vi "Sensor X Facade.vi"(0 "Data In":T5, 2 "Display State In":T3, 3 "Container State":T4) -> (6 "Data Out":T5, 7 "Display State Out":T3, 8 "Action":T2)   [LabVIEW 2013, in "Sensor X.xctl"]
uses:
  Sensor X.xctl
  Sensor X Data.ctl
  lib/Data Access Objects/Sensors/Sensor DAO Class.lvclass
  <vilib>/_xctls/Container State.ctl
  Sensor X State.ctl
  <vilib>/_xctls/Action.ctl
  Sensor Metadata.ctl
  lib/Data Access Objects/Sensors/Sensor DAO Class.lvclass/Sensor DAO Class.ctl
  <vilib>/_xctls/XControlSupport.lvlib
panel:
  in  "Sensor Metadata":T1
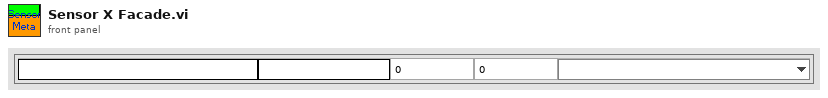
[diagram p1: front panel]
types:
  T1 = typedef "Sensor Metadata.ctl" = cluster{"Name":string, "Units":string, "Sensitivity":dbl, "Multiplier":dbl, "Excitation":u16}
  T2 = typedef "XControlSupport.lvlib/Action.ctl" = cluster{"Data Changed?":bool, "State Changed?":bool, "Action Name":string}
  T3 = typedef "Sensor X.xctl/Sensor X State.ctl" = cluster{"Volt Channels":string[]}
  T4 = typedef "XControlSupport.lvlib/Container State.ctl" = cluster{"Indicator?":bool, "Run Mode?":bool, " Refnum":refnum<vi>}
  T5 = typedef "Sensor X.xctl/Sensor X Data.ctl" = refnum<class "Sensor DAO Class.lvclass">
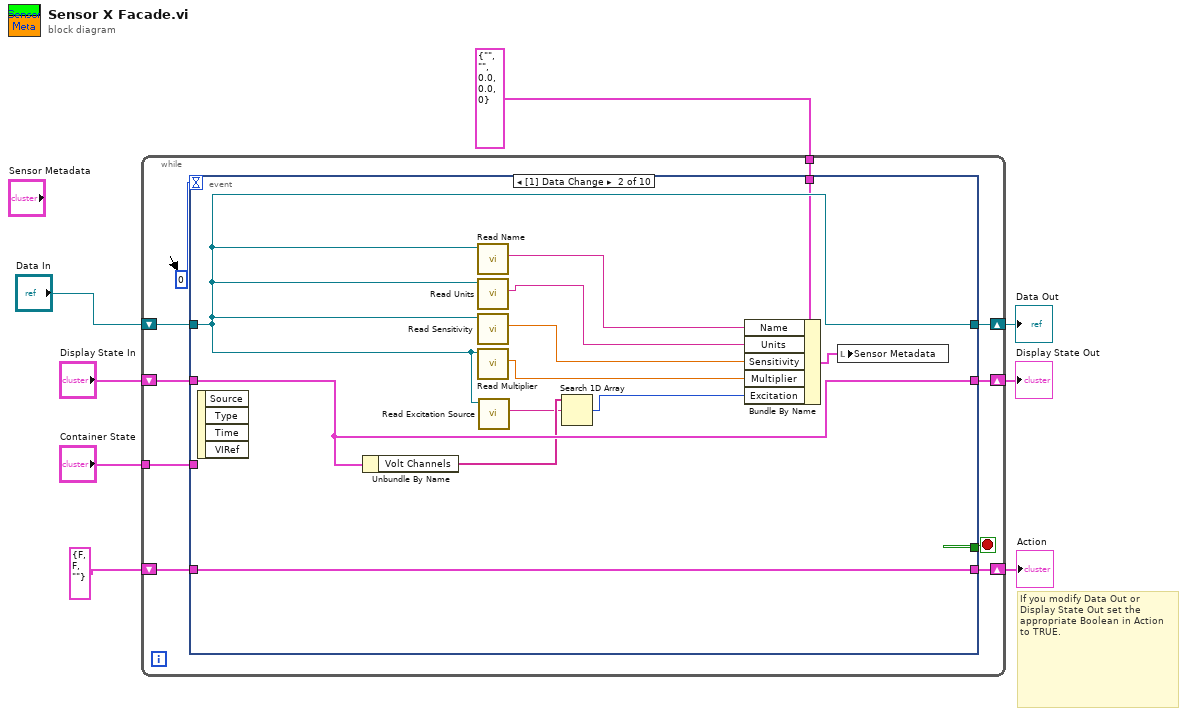
[diagram p0: block diagram]
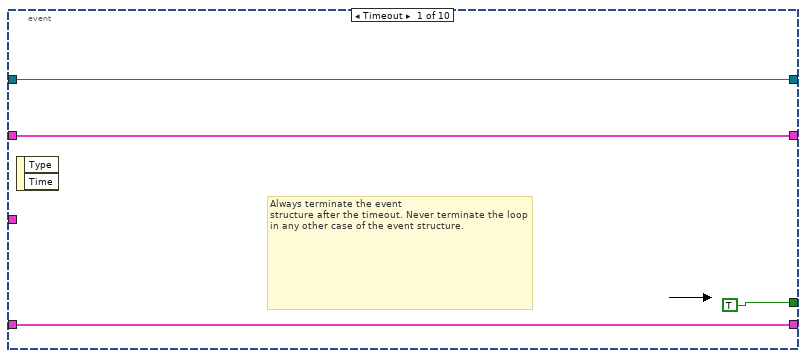
[diagram p2: hidden frame]
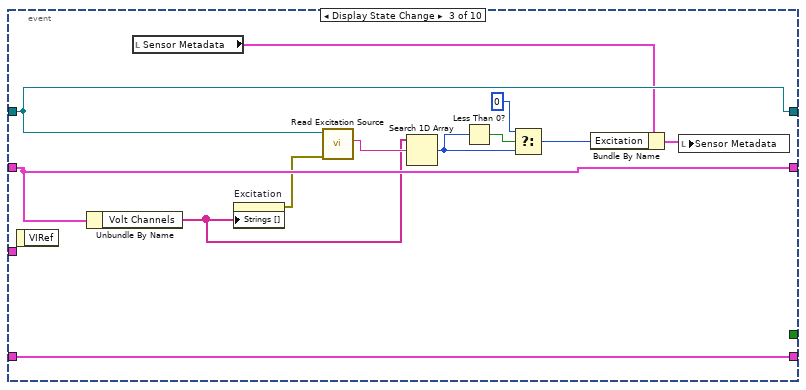
[diagram p3: hidden frame]
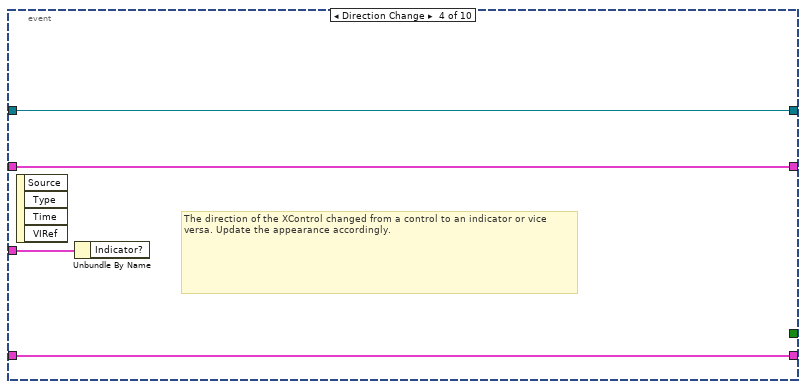
[diagram p4: hidden frame]
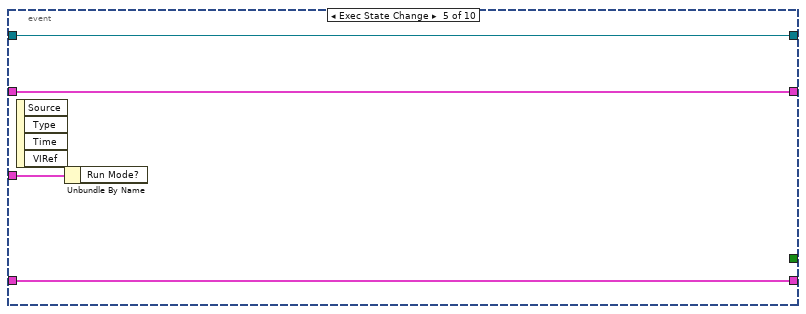
[diagram p5: hidden frame]
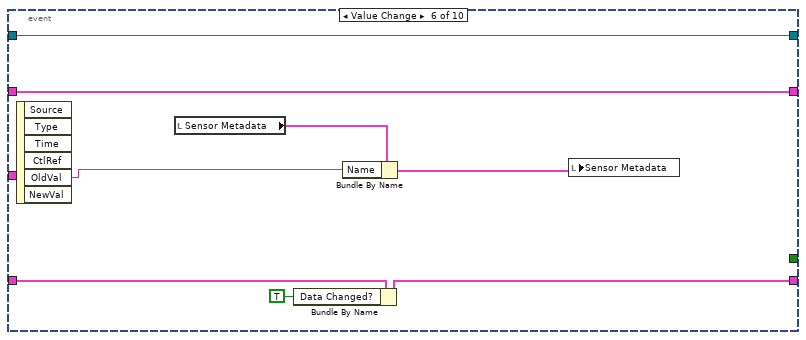
[diagram p6: hidden frame]
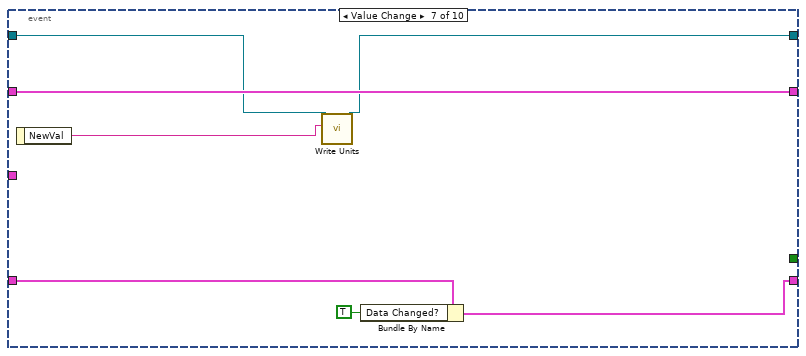
[diagram p7: hidden frame]
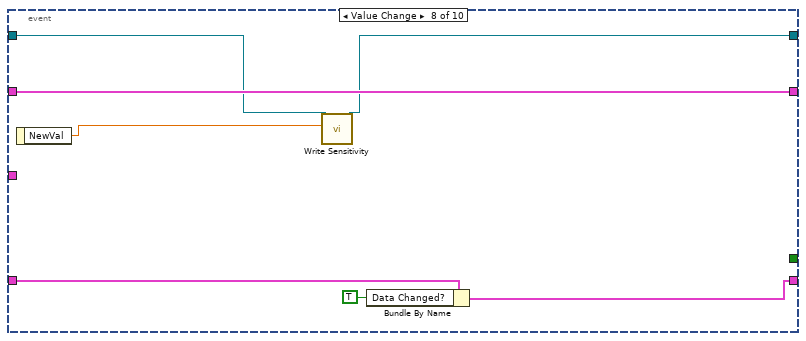
[diagram p8: hidden frame]
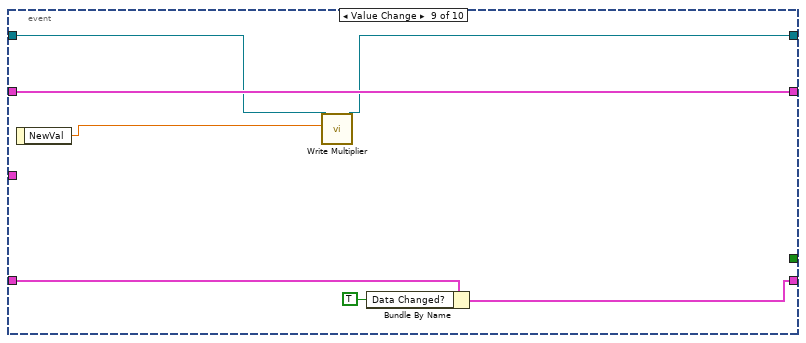
[diagram p9: hidden frame]
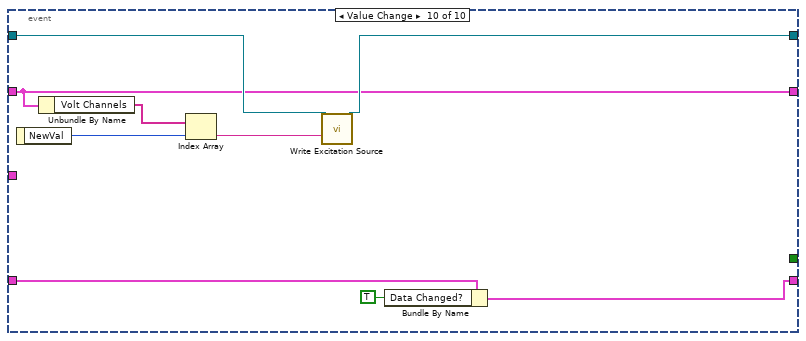
[diagram p10: hidden frame]
diagram:
  # "If you modify Data Out or\nDisplay State Out set the\nappropriate Boolean in Action\nto TRUE."
  n1 = while {
    shift-right: [w17] -> w5
    shift-left: "Display State In" -> [w18]
    tunnel: "Container State" -> [w14]
    shift-right: [w12] -> w8
    shift-left: "Data In" -> [w13]
    shift-right: [w10] -> w3
    shift-left: T2 {"Data Changed?"=FALSE, "State Changed?"=FALSE, "Action Name"=""} ("Action") -> [w11]
    tunnel: T1 {"Name"="", "Units"="", "Sensitivity"=0.0, "Multiplier"=0.0, "Excitation"=0} ("Sensor Metadata") -> [w9]
    stop <- w16 stop-if-true
    n2 = event shown="[1] Data Change" {
      selector: _ -> [_ _ _ _ _ _ _ _ _ _]
      dyn-events: _ -> [_ _ _ _ _ _ _ _ _ _]
      timeout: 0 -> [_ _ _ _ _ _ _ _ _ _]
      tunnel: w18 -> [w20 w27 w43 w49 w53 w62 w69 w76 w83 w89]
      tunnel: [w20 w27 w43 w49 w53 w62 w69 w76 w83 w89] -> w17
      tunnel: [TRUE _ _ _ _ _ _ _ _ _] -> w16
      tunnel: w14 -> [_ _ _ w50 w54 _ _ _ _ _]
      tunnel: w13 -> [w19 w33 w44 w48 w52 w61 w68 w75 w82 w92]
      tunnel: [w19 w33 w44 w48 w52 w61 w66 w74 w81 w91] -> w12
      tunnel: [w21 w34 w46 w47 w51 w56 w63 w70 w77 w84] -> w10
      tunnel: w11 -> [w21 w34 w46 w47 w51 w60 w64 w71 w78 w85]
      tunnel: w9 -> [_ w23 _ _ _ _ _ _ _ _]
      event Timeout {
        # "Always terminate the event\nstructure after the timeout. Never terminate the loop in any other case of the event structure."
        n3 = event-data() -> ()  [unwired: 1 in, 2 out]
      }
      event Data Change {
        n4 = event-data() -> ()  [unwired: 1 in, 4 out]
        n5 = Unbundle By Name(w27) -> ("Volt Channels"=w25:string[])
        n6 = call "Read Name.vi"("Sensor DAO Class in"=w33) -> ("Name"=w32:string)  [unwired: 8 in, 2 out]
        n7 = call "Read Units.vi"("Sensor DAO Class in"=w33) -> ("Units"=w31:string)  [unwired: 8 in, 2 out]
        n8 = call "Read Sensitivity.vi"("Sensor DAO Class in"=w33) -> ("Sensitivity"=w30:dbl)  [unwired: 8 in, 2 out]
        n9 = call "Read Multiplier.vi"("Sensor DAO Class in"=w33) -> ("Multiplier"=w29:dbl)  [unwired: 8 in, 2 out]
        n10 = call "Read Excitation Source.vi"("Sensor DAO Class in"=w33) -> ("Excitation Source"=w24:string)  [unwired: 8 in, 2 out]
        n11 = Search 1D Array(1D array=w25, element=w24) -> (index of element=w26:i32)  [unwired: 1 in]
        n12 = Bundle By Name(cluster=w23, "Name"=w32, "Units"=w31, "Sensitivity"=w30, "Multiplier"=w29, "Excitation"=w26) -> (w28:T1)
        n13 = local write "Sensor Metadata"(w28) -> ()
      }
      event Display State Change {
        n14 = event-data() -> ()  [unwired: 1 in, 1 out]
        n15 = Unbundle By Name(w43) -> ("Volt Channels"=w40:string[])
        n16 = local read "Sensor Metadata"() -> (w42:T1)
        n17 = property on="Excitation" class="Ring (strict)"("Strings []"=w40) -> (error out=w39:errorcluster)  [unwired: 2 in, 1 out]
        n18 = call "Read Excitation Source.vi"("error in (no error)"=w39, "Sensor DAO Class in"=w44) -> ("Excitation Source"=w45:string)  [unwired: 7 in, 2 out]
        n19 = Search 1D Array(1D array=w40, element=w45) -> (index of element=w37:i32)  [unwired: 1 in]
        n20 = Less Than 0?(x=w37) -> (x < 0?=w38:bool)
        n21 = Select(t=0, s=w38, f=w37) -> (s? t:f=w36:i32)
        n22 = Bundle By Name(cluster=w42, "Excitation"=w36) -> (w41:T1)
        n23 = local write "Sensor Metadata"(w41) -> ()
      }
      event Direction Change {
        # "The direction of the XControl changed from a control to an indicator or vice versa. Update the appearance accordingly."
        n24 = event-data() -> ()  [unwired: 1 in, 4 out]
        n25 = Unbundle By Name(w50) -> ()  [unwired: 1 out]
      }
      event Exec State Change {
        n26 = event-data() -> ()  [unwired: 1 in, 4 out]
        n27 = Unbundle By Name(w54) -> ()  [unwired: 1 out]
      }
      event Value Change {
        n28 = event-data() -> ("OldVal"=w57:string)  [unwired: 1 in, 5 out]
        n29 = local read "Sensor Metadata"() -> (w58:T1)
        n30 = Bundle By Name(cluster=w60, "Data Changed?"=TRUE) -> (w56:T2)
        n31 = Bundle By Name(cluster=w58, "Name"=w57) -> (w59:T1)
        n32 = local write "Sensor Metadata"(w59) -> ()
      }
      event Value Change {
        n33 = event-data() -> ("NewVal"=w67:string)  [unwired: 1 in]
        n34 = call "Write Units.vi"("Units"=w67, "Sensor DAO Class in"=w68) -> ("Sensor DAO Class out"=w66:T5)  [unwired: 8 in, 1 out]
        n35 = Bundle By Name(cluster=w64, "Data Changed?"=TRUE) -> (w63:T2)
      }
      event Value Change {
        n36 = event-data() -> ("NewVal"=w73:dbl)  [unwired: 1 in]
        n37 = call "Write Sensitivity.vi"("Sensitivity"=w73, "Sensor DAO Class in"=w75) -> ("Sensor DAO Class out"=w74:T5)  [unwired: 8 in, 1 out]
        n38 = Bundle By Name(cluster=w71, "Data Changed?"=TRUE) -> (w70:T2)
      }
      event Value Change {
        n39 = event-data() -> ("NewVal"=w80:dbl)  [unwired: 1 in]
        n40 = call "Write Multiplier.vi"("Multiplier"=w80, "Sensor DAO Class in"=w82) -> ("Sensor DAO Class out"=w81:T5)  [unwired: 8 in, 1 out]
        n41 = Bundle By Name(cluster=w78, "Data Changed?"=TRUE) -> (w77:T2)
      }
      event Value Change {
        n42 = event-data() -> ("NewVal"=w87:u16)  [unwired: 1 in]
        n43 = Unbundle By Name(w89) -> ("Volt Channels"=w88:string[])
        n44 = Index Array(array=w88, index=w87) -> (element=w90:string)
        n45 = call "Write Excitation Source.vi"("Excitation Source"=w90, "Sensor DAO Class in"=w92) -> ("Sensor DAO Class out"=w91:T5)  [unwired: 8 in, 1 out]
        n46 = Bundle By Name(cluster=w85, "Data Changed?"=TRUE) -> (w84:T2)
      }
    }
  }
  "Display State Out" <- w5
  "Data Out" <- w8
  "Action" <- w3
